vi "Read Config.lvclass.vi"(8 "error in (no error)":errorcluster, 11 "DelayLine in":refnum<class "DelayLine.lvclass">) -> (0 "error out":errorcluster, 2 "Config.lvclass":refnum<class "Config.lvclass">, 3 "DelayLine out":refnum<class "DelayLine.lvclass">)   [LabVIEW 2015]
uses:
  DelayLine.lvclass
  Config/Config.lvclass
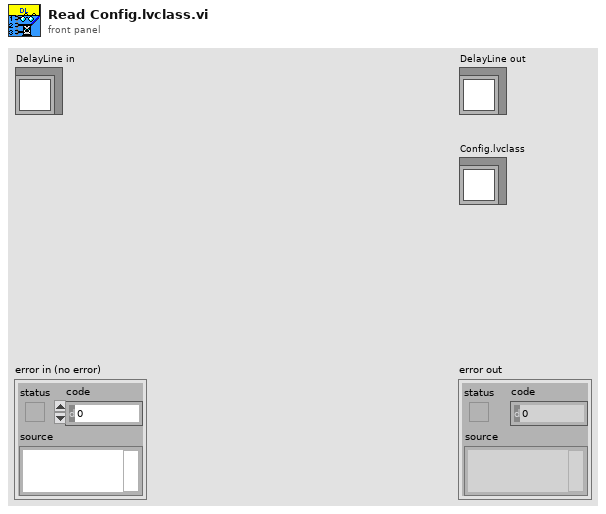
[diagram p1: front panel]
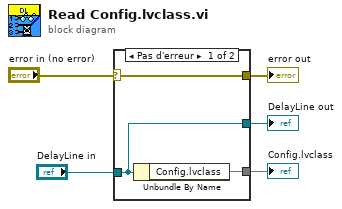
[diagram p0: block diagram]
diagram:
  n1 = case shown="Pas d'erreur" "error in (no error)" {
    selector: "error in (no error)" -> [w8 w9]
    tunnel: [w8 w9] -> w4
    tunnel: [w7 w10] -> w2
    tunnel: "DelayLine in" -> [w7 w10]
    tunnel: [w6 _] -> w1
    frame No Error {
      n2 = Unbundle By Name(w7) -> ("Config.lvclass"=w6)
    }
    frame Error {
    }
  }
  "error out" <- w4
  "DelayLine out" <- w2
  "Config.lvclass" <- w1
